vi "Main_Temperature.vi"() -> ()   [LabVIEW 2021]
uses:
  <vilib>/Analysis/NI_AALBase.lvlib
  Selector.ctl
  <vilib>/Analysis/baseanly.llb/Mean (DBL).vi
  <vilib>/DAQmx/read.llb/DAQmx Read (Analog 1D DBL 1Chan NSamp).vi
  <vilib>/Utility/file.llb/Write Delimited Spreadsheet (string).vi
  <vilib>/DAQmx/create/channels.llb/DAQmx Create Channel (AI-Voltage-Basic).vi
  <vilib>/DAQmx/configure/timing.llb/DAQmx Timing (Sample Clock).vi
panel:
  out "Iteración":i32
  in  "Save Data":bool
  in  "File Path":path
  out "Temp [Graph]":dbl(graph)
  in  "Stop":bool
  out "Temp":dbl
  # "Método de conexión:\n\nVs al puerto 5V de MyDAQ [17]\nVout conectado al puerto AI 0+ [11]\nGround debe de conectarse a AGND [1] y otro cable \nconectado al puerto AI0- [12] | IMPORTANTE |\n\nNota: Si el sensor se calienta significa que hicieron\nla conexión al revés, deben de tener cuidado con eso."
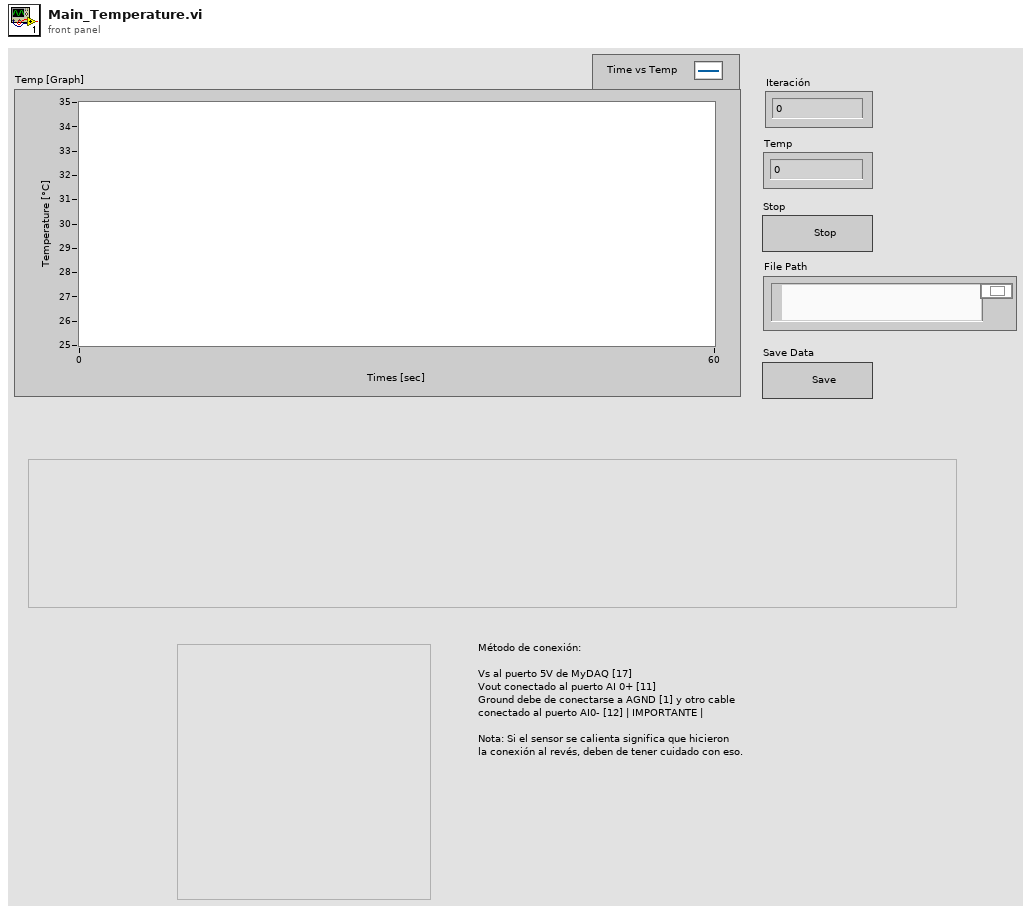
[diagram p1: front panel]
types:
  T1 = typedef "Selector.ctl" = enum16{"Stand By", "Path", "Measurement", "Wait"}
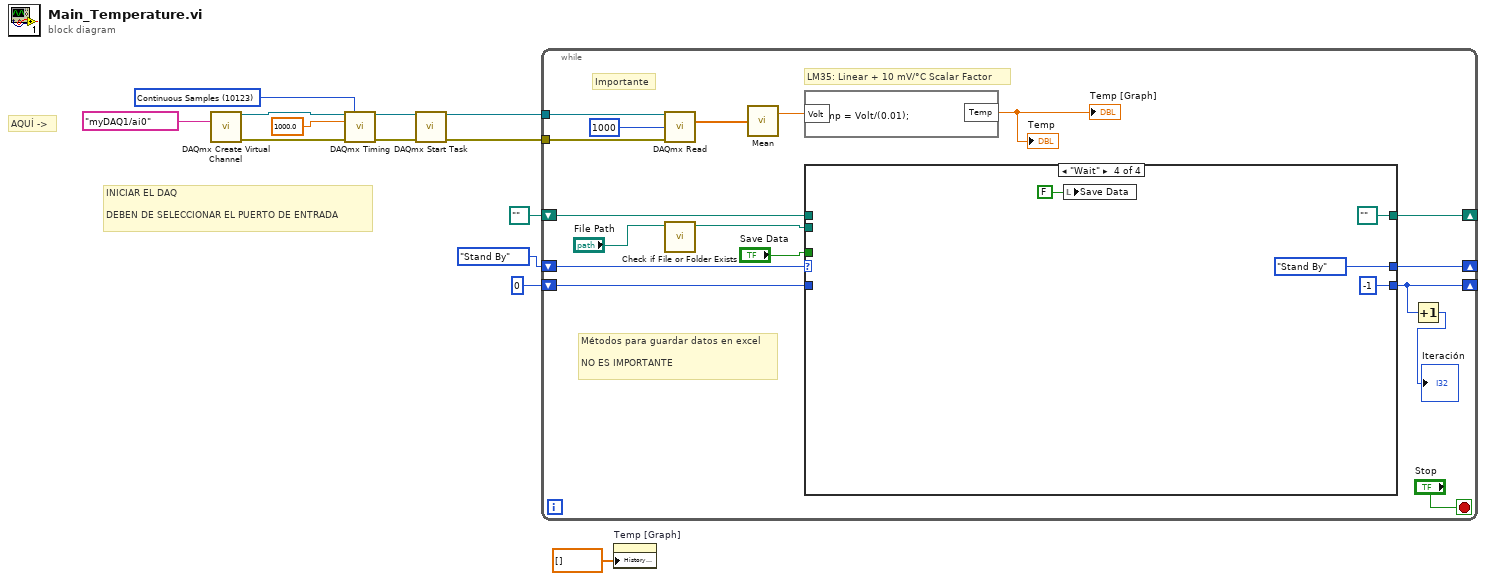
[diagram p0: block diagram]
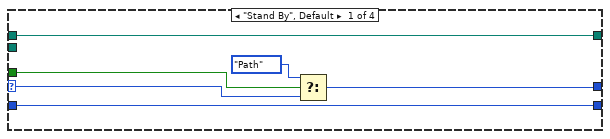
[diagram p2: hidden frame]
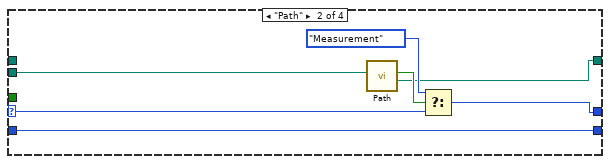
[diagram p3: hidden frame]
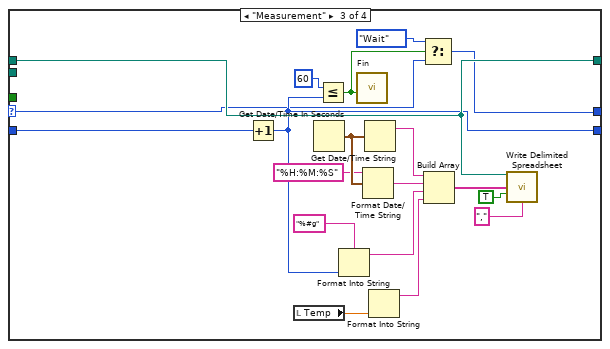
[diagram p4: hidden frame]
diagram:
  w10 = 10123 items=["Finite Samples"=10178, "Continuous Samples"=10123, "Hardware Timed Single Point"=12522] ("sample mode")
  # "AQUÍ ->"
  # "INICIAR EL DAQ\n\nDEBEN DE SELECCIONAR EL PUERTO DE ENTRADA"
  n1 = call-poly <vilib>:"DAQmx Create Virtual Channel.vi"("physical channels"=tag "myDAQ1/ai0") -> ("task out"=w4:refnum<k21>, "error out"=w3:errorcluster)  [unwired: 13 in]
  n2 = call-poly <vilib>:"DAQmx Timing.vi"("task/channels in"=w4, "sample mode"=w10, "rate"=1000.0, "error in"=w3) -> ("task out"=w8:refnum<k21>, "error out"=w7:errorcluster)  [unwired: 10 in]
  n3 = call <vilib>:"DAQmx Start Task.vi"("task/channels in"=w8, "error in"=w7) -> ("task out"=w6:refnum<k21>, "error out"=w5:errorcluster)  [unwired: 12 in]
  n4 = while {
    tunnel: w6 -> [w30]
    tunnel: w5 -> [w29]
    shift-right: [w21] -> _
    shift-left: Selector."Stand By" -> [w22]
    shift-right: [w15] -> _
    shift-left: 0 -> [w16]
    shift-right: [w18] -> _
    shift-left: path "" ("appended path") -> [w19]
    stop <- "Stop" stop-if-true
    # "Métodos para guardar datos en excel\n\nNO ES IMPORTANTE"
    # "Importante"
    # "LM35: Linear + 10 mV/°C Scalar Factor"
    n5 = call-poly <vilib>:"DAQmx Read.vi"("task/channels in"=w30, "number of samples per channel"=1000, "error in"=w29) -> ("data"=w28:dbl[])  [unwired: 10 in, 2 out]
    n6 = call <vilib>:"Check if File or Folder Exists.vi"("path"="File Path") -> ("dup path"=w20:path)  [unwired: 8 in, 2 out]
    n7 = call-poly <vilib>:"Mean.vi"("X"=w28) -> ("mean"=w27:dbl)  [unwired: 1 out]
    n8 = formula code="Temp = Volt/(0.01);"("Volt"=w27) -> ("Temp"=→"Temp" →"Temp [Graph]":dbl)
    n9 = case shown="\"Wait\"" w22 {
      selector: w22 -> [w34 w41 w47 _]
      tunnel: "Save Data" -> [w35 _ _ _]
      tunnel: [w33 w40 w45 Selector."Stand By"] -> w21
      tunnel: w20 -> [_ w43 _ _]
      tunnel: w16 -> [w32 w38 w58 _]
      tunnel: [w32 w38 w49 -1] -> w15
      tunnel: w19 -> [w31 _ w50 _]
      tunnel: [w31 w37 w50 path "" ("appended path")] -> w18
      frame "Stand By", Default {
        n10 = Select(t=Selector."Path", s=w35, f=w34) -> (s? t:f=w33:T1)
      }
      frame "Path" {
        n11 = call "Path.vi"("selected path"=w43) -> ("Boolean"=w42:bool, "appended path"=w37:path)  [unwired: 8 in]
        n12 = Select(t=Selector."Measurement", s=w42, f=w41) -> (s? t:f=w40:T1)
      }
      frame "Measurement" {
        n13 = Increment(x=w58) -> (x+1=w49:i32)
        n14 = local read "Temp"() -> (w59:dbl)
        n15 = Get Date/Time In Seconds() -> (seconds since 1Jan1904=w62:timestamp)
        n16 = Less Or Equal?(x=60, y=w49) -> (x <= y?=w44:bool)
        n17 = Format Into String(format string="%#g", w49) -> (resulting string=w52:string)  [unwired: 2 in, 1 out]
        n18 = call "Fin"("Enable"=w44) -> ()  [unwired: 9 in, 2 out]
        n19 = Format Date/Time String(time format string (%c)="%H:%M:%S", seconds (now)=w62) -> (date/time string=w53:string)  [unwired: 1 in]
        n20 = Get Date/Time String(seconds (now)=w62) -> (date string=w54:string)  [unwired: 2 in, 1 out]
        n21 = Format Into String(w59) -> (resulting string=w51:string)  [unwired: 3 in, 1 out]
        n22 = Select(t=Selector."Wait", s=w44, f=w47) -> (s? t:f=w45:T1)
        n23 = Build Array(w54, w53, w52, w51) -> (w55:string[])
        n24 = call-poly <vilib>:"Write Delimited Spreadsheet.vi"("file path (dialog if empty)"=w50, "1D data"=w55, "append to file? (new file:F)"=TRUE, "delimiter (\\t)"="," ("delimiter (\\t)")) -> ()  [unwired: 10 in, 2 out]
      }
      frame "Wait" {
        n25 = local write "Save Data"(FALSE ("Save Data")) -> ()
      }
    }
    n26 = Increment(x=w15) -> (x+1=→"Iteración":i32)
  }
  n27 = property on="Temp [Graph]" class="WFChart (strict)"("History Data"=dbl[] []) -> ()  [unwired: 2 in, 2 out]
